vi "Configure Measurement Mode.vi"(5 "Enable Current Measurement (T: Enable)":bool=TRUE, 6 "Enable Resistance Measurement (F: Disable)":bool, 7 "Enable Voltage Measurement (T: Enable)":bool=TRUE, 8 "error in (no error)":errorcluster, 10 "Channel (0: Channel 1)":i32(ring) items=["Channel 1", "Channel 2"], 11 "VISA resource name":refnum<visa-resource-name>) -> (0 "error out":errorcluster, 3 "VISA resource name out":refnum<visa-resource-name>)   [LabVIEW 2026, in "Agilent B2900 Series.lvlib"]
doc: "Configures the specified measurement functions to be enabled or disabled. \nTo enable measurement channel, call Enable Output.vi"
uses:
  Agilent B2900 Series.lvlib
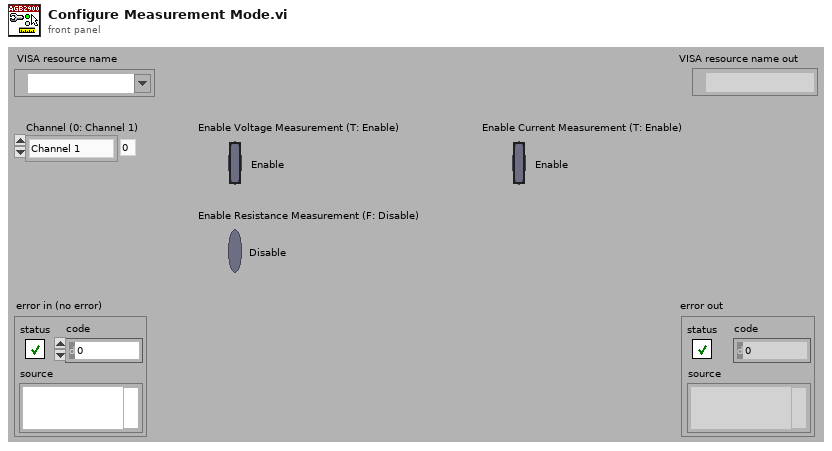
[diagram p1: front panel]
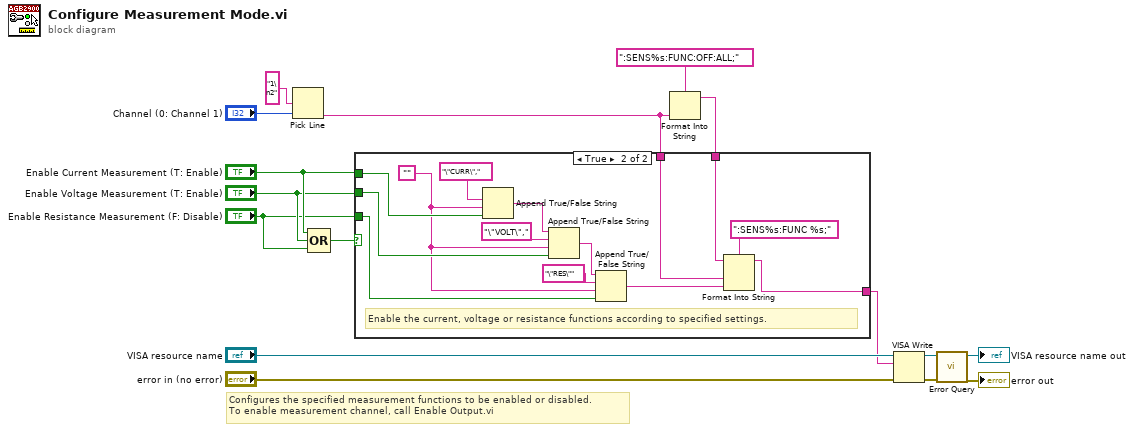
[diagram p0: block diagram]
diagram:
  # "Configures the specified measurement functions to be enabled or disabled. \nTo enable measurement channel, call Enable Output.vi"
  n1 = Pick Line(multi-line string="1\n2" ("string (\"\")"), line index="Channel (0: Channel 1)") -> (output string=w2:string)  [unwired: 1 in]
  n2 = Compound Arithmetic op=OR("Enable Current Measurement (T: Enable)", "Enable Voltage Measurement (T: Enable)", "Enable Resistance Measurement (F: Disable)") -> (w10:bool)
  n3 = Format Into String(format string=":SENS%s:FUNC:OFF:ALL;", w2) -> (resulting string=w3:string)  [unwired: 2 in, 1 out]
  n4 = case shown="True" w10 {
    tunnel: "Enable Current Measurement (T: Enable)" -> [_ w31]
    tunnel: "Enable Voltage Measurement (T: Enable)" -> [_ w28]
    tunnel: "Enable Resistance Measurement (F: Disable)" -> [_ w24]
    tunnel: w2 -> [_ w21]
    tunnel: w3 -> [w17 w20]
    tunnel: [w17 w19] -> w1
    frame False {
    }
    frame True {
      w23 = ""
      # "Enable the current, voltage or resistance functions according to specified settings."
      n5 = Append True/False String(1:w31, 2:w23, 3:"\"CURR\",") -> (0:w26:string)  [unwired: 1 in]
      n6 = Append True/False String(1:w28, 2:w23, 3:"\"VOLT\",", 4:w26) -> (0:w27:string)
      n7 = Append True/False String(1:w24, 2:w23, 3:"\"RES\"", 4:w27) -> (0:w18:string)
      n8 = Format Into String(format string=":SENS%s:FUNC %s;", initial string=w20, w21, w18) -> (resulting string=w19:string)  [unwired: 1 in, 1 out]
    }
  }
  n9 = VISA Write(VISA resource name="VISA resource name", write buffer=w1, error in (no error)="error in (no error)") -> (VISA resource name out=w14:refnum<visa-resource-name>, error out=w13:errorcluster)  [unwired: 1 out]
  n10 = call "Error Query.vi"("error in (no error)"=w13, "VISA resource name"=w14) -> ("error out"=→"error out":errorcluster, "VISA resource name out"=→"VISA resource name out":refnum<visa-resource-name>)  [unwired: 6 in, 2 out]
